vi "FGV milisec (subVI).vi"() -> (3 "Elased Time (ms)":u32)   [LabVIEW 2018, in "Application.lvlib"]
uses:
  Application.lvlib
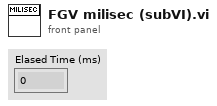
[diagram p1: front panel]
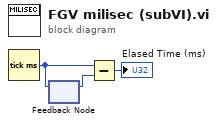
[diagram p0: block diagram]
diagram:
  n1 = Tick Count (ms)() -> (millisecond timer value=w2:u32)
  n2 = feedback-in #1(w2) -> ()
  n3 = feedback #1() -> (w3:u32)  [unwired: 1 in]
  n4 = Subtract(x=w2, y=w3) -> (x-y=→"Elased Time (ms)":u32)
